vi "create_save_dir_and_fn.vi"(8 "scn_iter":i32, 9 "sample":string="testSample", 10 "Experiment":string="testExp", 11 "data folder":path=path "Z:/11 Setups/04 NOPA TA/01 Data") -> (3 "Path":path)   [LabVIEW 2019]
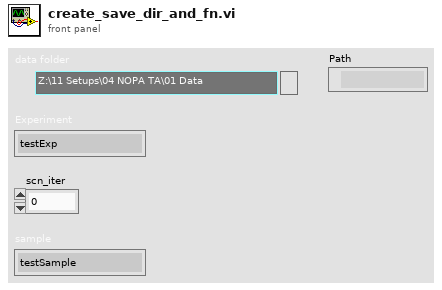
[diagram p1: front panel]
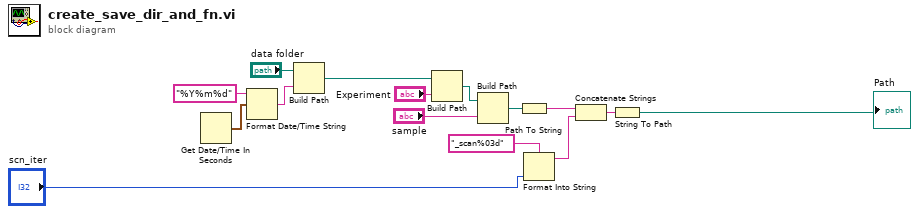
[diagram p0: block diagram]
diagram:
  n1 = Get Date/Time In Seconds() -> (seconds since 1Jan1904=w8:timestamp)
  n2 = Format Date/Time String(time format string (%c)="%Y%m%d", seconds (now)=w8) -> (date/time string=w6:string)  [unwired: 1 in]
  n3 = Build Path(base path="data folder", name or relative path=w6) -> (appended path=w5:path)
  n4 = Build Path(base path=w5, name or relative path="Experiment") -> (appended path=w3:path)
  n5 = Build Path(base path=w3, name or relative path="sample") -> (appended path=w13:path)
  n6 = Path To String(path=w13) -> (string=w9:string)
  n7 = Format Into String(format string="_scan%03d" ("initial string"), "scn_iter") -> (resulting string=w12:string)  [unwired: 2 in, 1 out]
  n8 = Concatenate Strings(w9, w12) -> (w10:string)
  n9 = String To Path(string=w10) -> (path=→"Path":path)
